vi "Render.vi"(8 "error in (no error)":errorcluster, 11 "IAmVIEW in":refnum<class "IAmVIEW.lvclass">) -> (0 "error out":errorcluster, 3 "IAmVIEW out":refnum<class "IAmVIEW.lvclass">)   [LabVIEW 2020, in "GLF.lvlib" / "IAmVIEW.lvclass"]
uses:
  IAmVIEW.lvclass
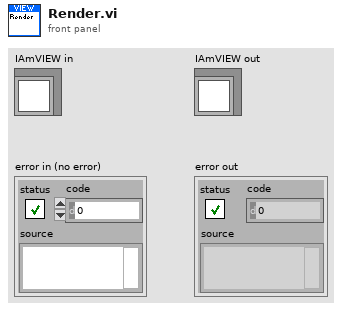
[diagram p1: front panel]
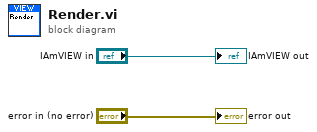
[diagram p0: block diagram]
diagram:
  "error out" <- "error in (no error)"
  "IAmVIEW out" <- "IAmVIEW in"
